vi "Module Queue FGV.vi"(8 "Error in":errorcluster, 9 "Queue name":string, 10 "Module Queue Actions":T1=enum."Get") -> (0 "error out":errorcluster, 3 "Queue out":refnum<queue>)   [LabVIEW 2018, in "Display Console.lvlib"]
doc: "To access module queue"
uses:
  Display Console.lvlib
  Module Queue Actions.ctl
  ctl/Module Message--cluster.ctl
  ctl/Module State--enum.ctl
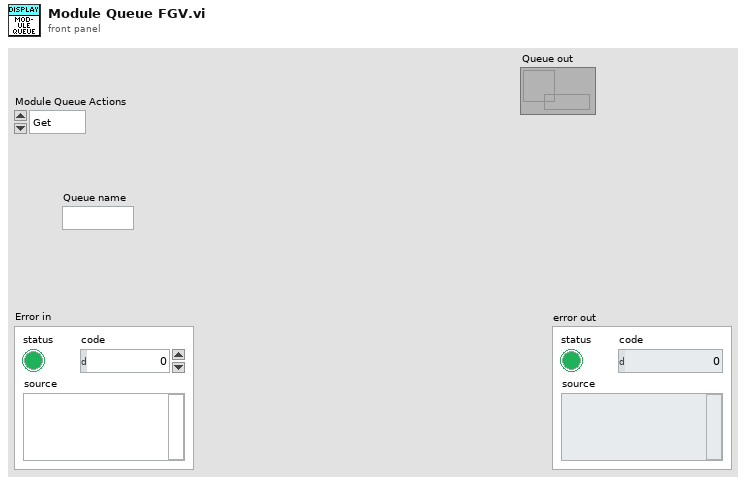
[diagram p1: front panel]
types:
  T1 = typedef "Display Console.lvlib/Module Queue Actions.ctl" = enum16{"Create", "Get", "Destroy"}
  T2 = typedef "Display Console.lvlib/Module Message--cluster.ctl" = cluster{"State":T3, "Data":variant}
  T3 = typedef "Display Console.lvlib/Module State--enum.ctl" = enum16{"Init", "Error", "Idle", "Close", "Card Read LED", "Update Message Screen", "Update Current Transaction", "Enable/disable controls"}
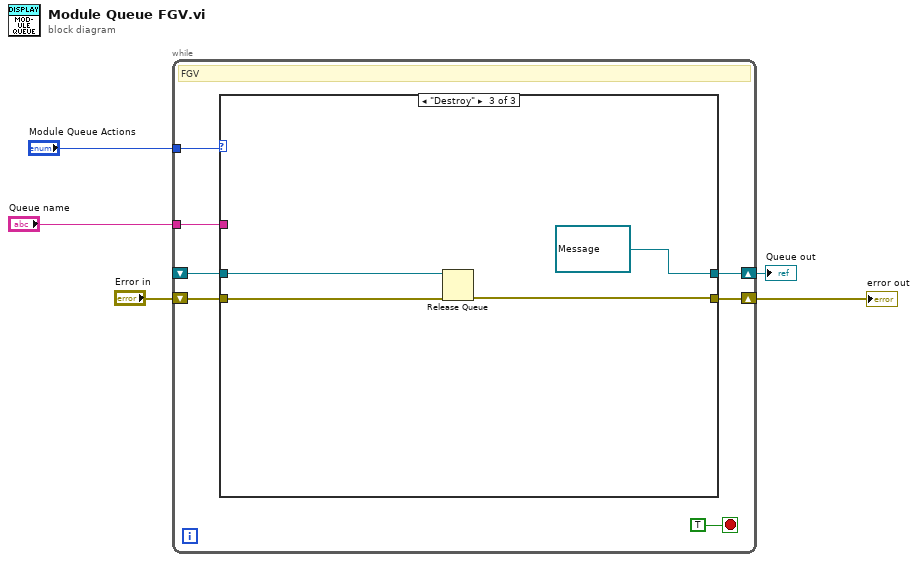
[diagram p0: block diagram]
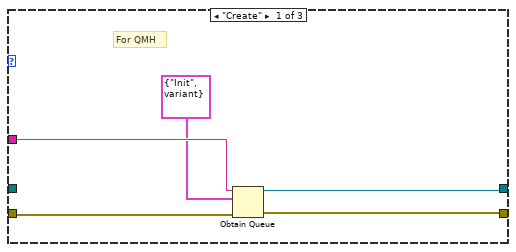
[diagram p2: hidden frame]
diagram:
  n1 = while {
    tunnel: "Module Queue Actions" -> [w12]
    shift-right: [w10] -> w1
    shift-left: _ -> [w9]
    shift-right: [w8] -> w4
    shift-left: "Error in" -> [w7]
    tunnel: "Queue name" -> [w6]
    stop <- TRUE stop-if-true
    # "FGV"
    n2 = case shown="\"Destroy\"" w12 {
      tunnel: [w17 w19 refnum<queue> refnum ("queue out")] -> w10
      tunnel: w9 -> [_ w19 w22]
      tunnel: [w16 w18 w23] -> w8
      tunnel: w7 -> [w14 w18 w21]
      tunnel: w6 -> [w15 _ _]
      frame "Create" {
        # "For QMH"
        n3 = Obtain Queue(name (unnamed)=w15, element data type=T2 {"State"=enum."Init", "Data"=variant} ("Message"), error in (no error)=w14) -> (queue out=w17:refnum<queue>, error out=w16:errorcluster)  [unwired: 2 in, 1 out]
      }
      frame "Get", Default {
      }
      frame "Destroy" {
        n4 = Release Queue(queue=w22, error in (no error)=w21) -> (error out=w23:errorcluster)  [unwired: 1 in, 2 out]
      }
    }
  }
  "error out" <- w4
  "Queue out" <- w1
